vi "controller disconnect.vi"(11 "controller 2":T1) -> ()   [LabVIEW 2016]
uses:
  Classes/Controller/Motion/A3200 Folder/A3200.lvclass
  Classes/Controller/Dispenser/Ultimus V2 Folder/Ultimus V2.lvclass
  Classes/Controller/I-O/NI-DAQ Folder/NI-DAQ.lvclass
  Classes/Controller/Motion/Motion Folder/Motion.lvclass
  Classes/Controller/I-O/I-O Folder/I-O.lvclass
  Classes/Controller/Dispenser/Dispenser Folder/Dispenser.lvclass
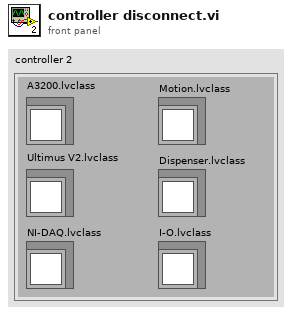
[diagram p1: front panel]
types:
  T1 = cluster{"A3200.lvclass":refnum<class "A3200.lvclass">, "Ultimus V2.lvclass":refnum<class "Ultimus V2.lvclass">, "NI-DAQ.lvclass":refnum<class "NI-DAQ.lvclass">, "Motion.lvclass":refnum<class "Motion.lvclass">, "I-O.lvclass":refnum<class "I-O.lvclass">, "Dispenser.lvclass":refnum<class "Dispenser.lvclass">}
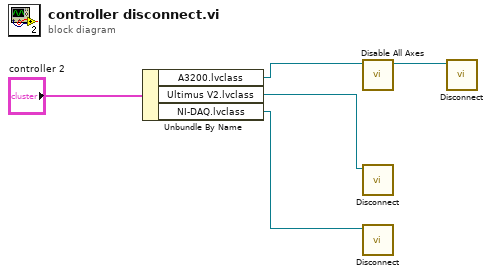
[diagram p0: block diagram]
diagram:
  n1 = Unbundle By Name("controller 2") -> ("A3200.lvclass"=w5:refnum<class "A3200.lvclass">, "Ultimus V2.lvclass"=w2:refnum<class "Ultimus V2.lvclass">, "NI-DAQ.lvclass"=w3:refnum<class "NI-DAQ.lvclass">)
  n2 = call-dynamic "Disable All Axes.vi"("Gantry in"=w5) -> ("Gantry out"=w4:refnum<class "A3200.lvclass">)  [unwired: 9 in, 1 out]
  n3 = call-dynamic "Disconnect.vi"("Ultimus V in"=w2) -> ()  [unwired: 9 in, 1 out]
  n4 = call-dynamic "Disconnect.vi"("I-O in"=w3) -> ()  [unwired: 9 in, 1 out]
  n5 = call-dynamic "Disconnect.vi"("Gantry in"=w4) -> ()  [unwired: 9 in, 1 out]
